vi "Encoder_to_Phi.vi"(11 "Encoder Output":i32) -> (3 "Output Angle":dbl)   [LabVIEW 2014]
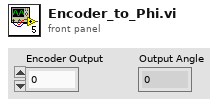
[diagram p1: front panel]
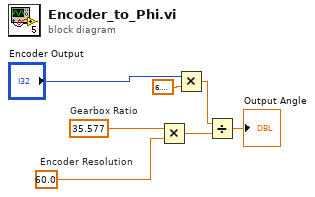
[diagram p0: block diagram]
diagram:
  w6 = 60.0  # Encoder Resolution
  w5 = 35.577  # Gearbox Ratio
  n1 = Multiply(x=w5, y=w6) -> (x*y=w4:dbl)
  n2 = Multiply(x="Encoder Output", y=6.283185307179586) -> (x*y=w3:dbl)
  n3 = Divide(x=w3, y=w4) -> (x/y=→"Output Angle":dbl)
